vi "Get Setpoint.vi"(8 "Current PID Setpoint":dbl, 11 "Level":dbl) -> (3 "Setpoint":dbl)   [LabVIEW 2014]
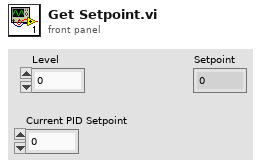
[diagram p1: front panel]
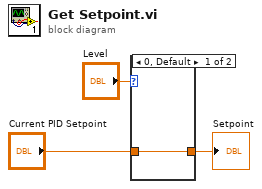
[diagram p0: block diagram]
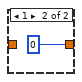
[diagram p2: hidden frame]
diagram:
  n1 = case shown="0, Default" "Level" {
    tunnel: [w4 0] -> w2
    tunnel: "Current PID Setpoint" -> [w4 _]
    frame 0, Default {
    }
    frame 1 {
    }
  }
  "Setpoint" <- w2
